vi "TestSpaceshipMove.vi"() -> ()   [LabVIEW 2017]
uses:
  Display/Display_mods.ctl
  Spaceship/Spaceship_mods.ctl
  <vilib>/Utility/inputDevices.llb/keyboardAcquire.vi
  <vilib>/Utility/inputDevices.llb/closeKeyboard.vi
panel:
  out "error out":errorcluster
  in  "stop":bool
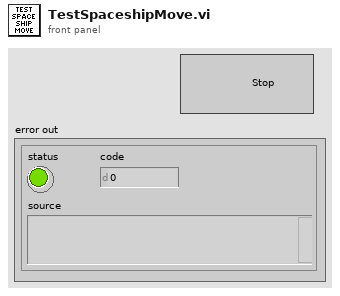
[diagram p1: front panel]
types:
  T1 = typedef "Spaceship_mods.ctl" = enum16{"Init", "Move", "Rotate", "Translate", "End"}
  T2 = typedef "Display_mods.ctl" = enum16{"Init", "GetBase", "DrawAster", "DrawShip", "Clear", "Close"}
  T3 = enum16{"0", "1", "2", "3", "4", "5", "6", "7", "8", "9", "A", "B", "C", "D", "E", "F", "G", "H", "I", "J", "K", "L", "M", "N", "O", "P", "Q", "R", "S", "T", "U", "V", "W", "X", "Y", "Z", "F1", "F2", "F3", "F4", "F5", "F6", "F7", "F8", "F9", "F10", "F11", "F12", "F13", "F14", "F15", "ADD", "BACK", "BACKSLASH", "CAPITAL", "COMMA", "DECIMAL", "DELETE", "DIVIDE", "DOWN", "END", "EQUALS", "ESCAPE", "GRAVE (`)", "HOME", "INSERT", "LBRACKET", "LCONTROL", "LEFT", "L ALT", "LSHIFT", "LWIN", "MINUS", "MULTIPLY", "NEXT", "NUMLOCK", "NUMPAD_0", "NUMPAD_1", "NUMPAD_2", "NUMPAD_3", "NUMPAD_4", "NUMPAD_5", "NUMPAD_6", "NUMPAD_7", "NUMPAD_8", "NUMPAD_9", "PAUSE", "PERIOD", "PRIOR (PG UP)", "RBRACKET", "RCONTROL", "RETURN", "RIGHT", "R ALT", "RSHIFT", "RWIN", "SCROLL", "SEMICOLON", "SLASH", "SPACE", "SUBTRACT", "TAB", "UP", "ENTER (num pad)", "' (quote)"}[]
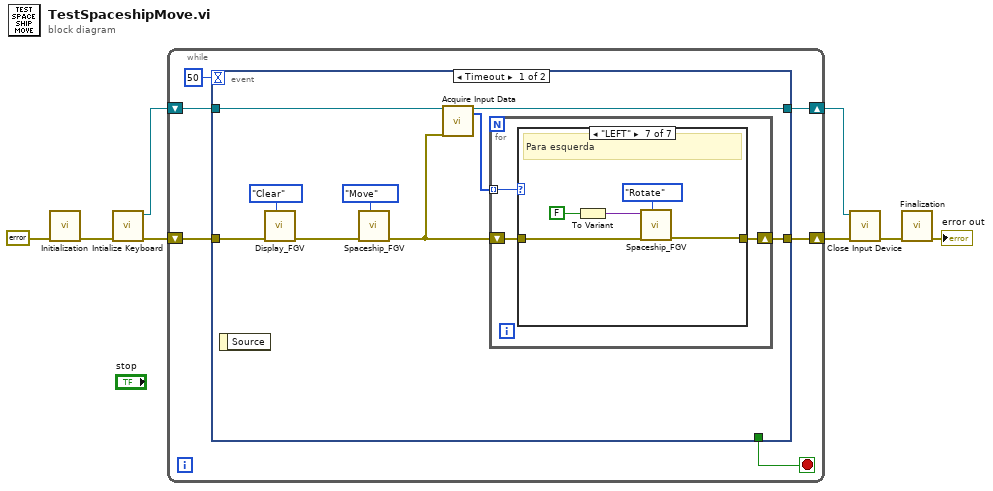
[diagram p0: block diagram]
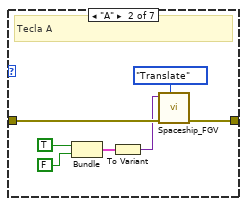
[diagram p3: hidden frame]
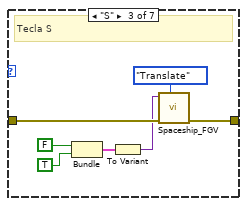
[diagram p4: hidden frame]
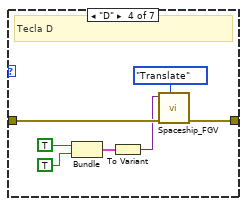
[diagram p5: hidden frame]
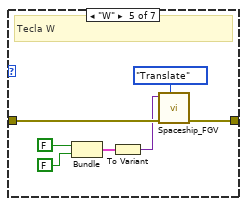
[diagram p6: hidden frame]
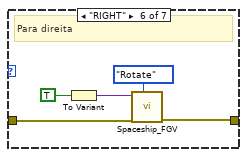
[diagram p7: hidden frame]
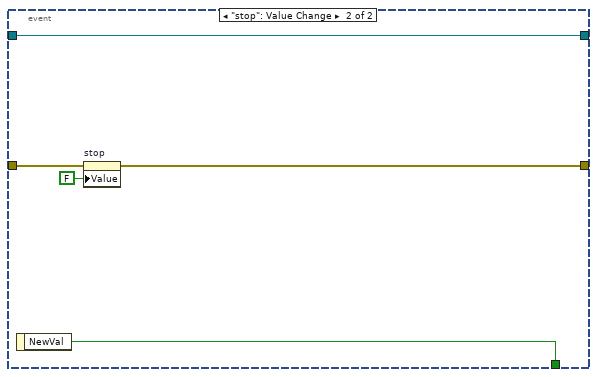
[diagram p8: hidden frame]
diagram:
  n1 = call "Initialization.vi"("error in"=errorcluster {"status"=FALSE, "code"=0, "source"=""}) -> ("error out"=w6:errorcluster)  [unwired: 10 in]
  n2 = call <vilib>:"Intialize Keyboard.vi"("error in (no error)"=w6) -> ("error out"=w5:errorcluster, "device ID"=w4:refnum<k1>)  [unwired: 9 in]
  n3 = while {
    shift-right: [w13] -> w3
    shift-left: w5 -> [w14]
    shift-right: [w9] -> w1
    shift-left: w4 -> [w10]
    stop <- w11 stop-if-true
    n4 = event shown="[0] Timeout" {
      selector: _ -> [_ _]
      dyn-events: _ -> [_ _]
      timeout: 50 -> [_ _]
      tunnel: w14 -> [w22 w68]
      tunnel: [w16 w67] -> w13
      tunnel: [_ w70] -> w11
      tunnel: w10 -> [w19 w66]
      tunnel: [w18 w66] -> w9
      event Timeout {
        n5 = event-data() -> ()  [unwired: 1 in, 1 out]
        n6 = call "Display_FGV.vi"("Display_mods"=Display_mods."Clear", "error in"=w22) -> ("error out"=w21:errorcluster)  [unwired: 8 in, 1 out]
        n7 = call "Spaceship_FGV.vi"("Spaceship_mods"=Spaceship_mods."Move", "error in"=w21) -> ("error out"=w17:errorcluster)  [unwired: 9 in]
        n8 = call-poly <vilib>:"Acquire Input Data.vi"("device ID"=w19, "error in (no error)"=w17) -> ("device ID"=w18:refnum<k1>, "keys pressed"=w15:T3)  [unwired: 15 in, 1 out]
        n9 = for {
          shift-right: [w25] -> w16
          shift-left: w17 -> [w26]
          tunnel: w15 -> [w24] mode=indexing
          n10 = case shown="\"LEFT\"" w24 {
            tunnel: w26 -> [w27 w33 w40 w47 w54 w59 w64]
            tunnel: [w27 w32 w39 w46 w53 w58 w63] -> w25
            frame "0", Default {
            }
            frame "A" {
              # "Tecla A"
              n11 = Bundle("stop"=TRUE, "stop"=FALSE) -> (w31:cluster{"stop":bool, "stop":bool})  [unwired: 1 in]
              n12 = To Variant(anything=w31) -> (Variant=w30:variant)
              n13 = call "Spaceship_FGV.vi"("Spaceship_mods"=Spaceship_mods."Translate", "error in"=w33, "DataIn"=w30) -> ("error out"=w32:errorcluster)  [unwired: 8 in]
            }
            frame "S" {
              # "Tecla S"
              n14 = Bundle("stop"=FALSE, "stop"=TRUE) -> (w38:cluster{"stop":bool, "stop":bool})  [unwired: 1 in]
              n15 = To Variant(anything=w38) -> (Variant=w37:variant)
              n16 = call "Spaceship_FGV.vi"("Spaceship_mods"=Spaceship_mods."Translate", "error in"=w40, "DataIn"=w37) -> ("error out"=w39:errorcluster)  [unwired: 8 in]
            }
            frame "D" {
              # "Tecla D"
              n17 = Bundle("stop"=TRUE, "stop"=TRUE) -> (w45:cluster{"stop":bool, "stop":bool})  [unwired: 1 in]
              n18 = To Variant(anything=w45) -> (Variant=w44:variant)
              n19 = call "Spaceship_FGV.vi"("Spaceship_mods"=Spaceship_mods."Translate", "error in"=w47, "DataIn"=w44) -> ("error out"=w46:errorcluster)  [unwired: 8 in]
            }
            frame "W" {
              # "Tecla W"
              n20 = Bundle("stop"=FALSE, "stop"=FALSE) -> (w52:cluster{"stop":bool, "stop":bool})  [unwired: 1 in]
              n21 = To Variant(anything=w52) -> (Variant=w51:variant)
              n22 = call "Spaceship_FGV.vi"("Spaceship_mods"=Spaceship_mods."Translate", "error in"=w54, "DataIn"=w51) -> ("error out"=w53:errorcluster)  [unwired: 8 in]
            }
            frame "RIGHT" {
              # "Para direita"
              n23 = To Variant(anything=TRUE ("stop")) -> (Variant=w57:variant)
              n24 = call "Spaceship_FGV.vi"("Spaceship_mods"=Spaceship_mods."Rotate", "error in"=w59, "DataIn"=w57) -> ("error out"=w58:errorcluster)  [unwired: 8 in]
            }
            frame "LEFT" {
              # "Para esquerda"
              n25 = To Variant(anything=FALSE ("stop")) -> (Variant=w62:variant)
              n26 = call "Spaceship_FGV.vi"("Spaceship_mods"=Spaceship_mods."Rotate", "error in"=w64, "DataIn"=w62) -> ("error out"=w63:errorcluster)  [unwired: 8 in]
            }
          }
        }
      }
      event "stop": Value Change {
        n27 = event-data() -> ("NewVal"=w70:bool)  [unwired: 1 in]
        n28 = property on="stop" class="Bool (strict)"(error in=w68, "Value"=FALSE ("Add")) -> (error out=w67:errorcluster)  [unwired: 1 in, 1 out]
      }
    }
  }
  n29 = call-poly <vilib>:"Close Input Device.vi"("error in (no error)"=w3, "device ID"=w1) -> ("error out"=w2:errorcluster)  [unwired: 8 in]
  n30 = call "Finalization.vi"("error in"=w2) -> ("error out"=→"error out":errorcluster)  [unwired: 10 in]
